vi "parseMotorStatus.vi"(8 "error in (no error)":errorcluster, 9 "inputStatus":u16, 11 "MotorController in":refnum<class "MotorController.lvclass">) -> (0 "error out":errorcluster, 2 "output cluster":T1, 3 "MotorController out":refnum<class "MotorController.lvclass">)   [LabVIEW 2017, in "MotorController.lvclass"]
uses:
  MotorController.lvclass
  MotorController.lvclass/MotorController.ctl
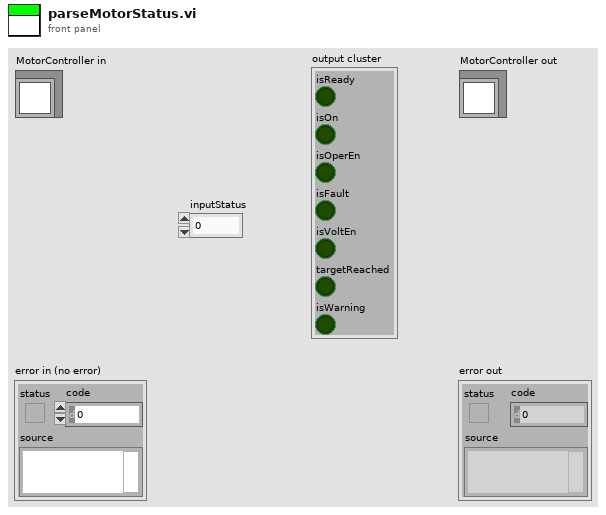
[diagram p1: front panel]
types:
  T1 = cluster{"isReady":bool, "isOn":bool, "isOperEn":bool, "isFault":bool, "isVoltEn":bool, "targetReached":bool, "isWarning":bool}
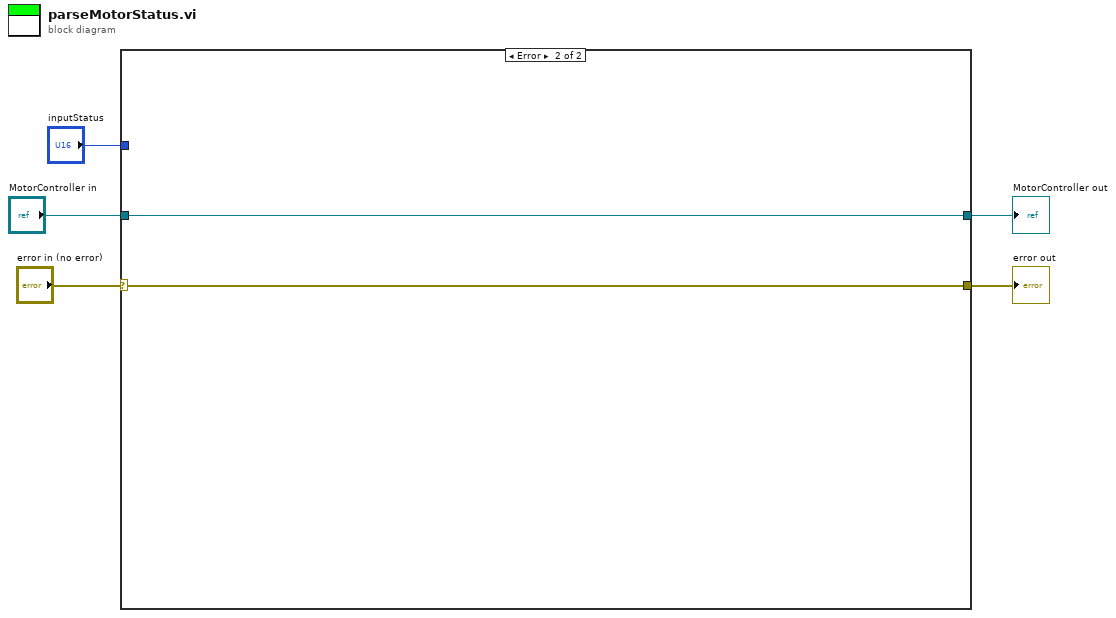
[diagram p0: block diagram]
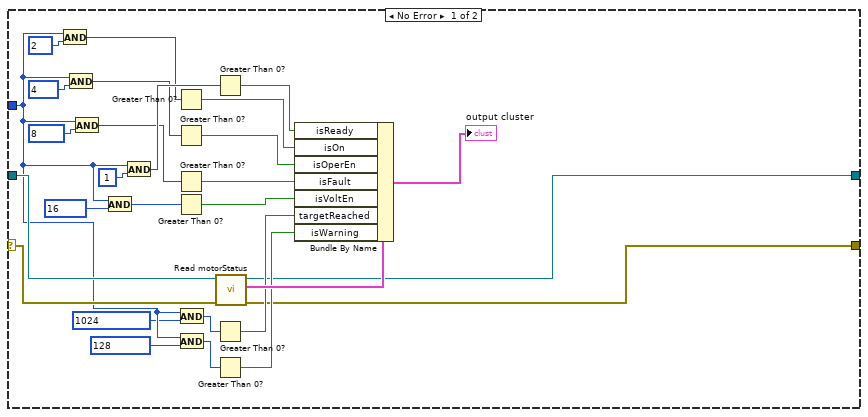
[diagram p2: hidden frame]
diagram:
  n1 = case shown="Error" "error in (no error)" {
    selector: "error in (no error)" -> [w32 w35]
    tunnel: [w8 w35] -> w4
    tunnel: [w7 w34] -> w2
    tunnel: "MotorController in" -> [w33 w34]
    tunnel: "inputStatus" -> [w29 _]
    frame No Error {
      n2 = And(x=w29, y=2) -> (x .and. y?=w25:i32)
      n3 = And(x=w29, y=4) -> (x .and. y?=w20:i32)
      n4 = And(x=w29, y=8) -> (x .and. y?=w24:i32)
      n5 = And(x=w29, y=16) -> (x .and. y?=w23:i32)
      n6 = And(x=w29, y=1) -> (x .and. y?=w27:i32)
      n7 = Greater Than 0?(x=w25) -> (x > 0?=w19:bool)
      n8 = Greater Than 0?(x=w20) -> (x > 0?=w17:bool)
      n9 = Greater Than 0?(x=w24) -> (x > 0?=w15:bool)
      n10 = Greater Than 0?(x=w23) -> (x > 0?=w11:bool)
      n11 = And(x=w29, y=1024) -> (x .and. y?=w21:i32)
      n12 = And(x=w29, y=128) -> (x .and. y?=w22:i32)
      n13 = Greater Than 0?(x=w27) -> (x > 0?=w26:bool)
      n14 = Greater Than 0?(x=w21) -> (x > 0?=w9:bool)
      n15 = Greater Than 0?(x=w22) -> (x > 0?=w10:bool)
      n16 = call "Read motorStatus.vi"("error in (no error)"=w32, "MotorController in"=w33) -> ("error out"=w8:errorcluster, "motorStatus"=w31:T1, "MotorController out"=w7:refnum<class "MotorController.lvclass">)  [unwired: 7 in]
      n17 = Bundle By Name(cluster=w31, "isReady"=w26, "isOn"=w19, "isOperEn"=w17, "isFault"=w15, "isVoltEn"=w11, "targetReached"=w9, "isWarning"=w10) -> (→"output cluster":T1)
    }
    frame Error {
    }
  }
  "error out" <- w4
  "MotorController out" <- w2
